vi "function2New.vi"   [LabVIEW 2016, in "Test.lvrbt"]
uses:
  Test.lvrbt
  <vilib>/NXT/Block Support/NXT_InputPort.ctl
  <vilib>/NXT/Hardware/Plugins/Tetrix DC Motor/TetrixDCMotorAddress.ctl
  <vilib>/NXT/NXTIO Xnodes/NXTIONodeSubVIs/TETRIX IO Move DC Motors.vi
  <vilib>/NXT/Dual Mode Library/Waits/Wait_EV3_Ultrasonic_Centimeter_Closer.vi
  <vilib>/NXT/NXTIO Xnodes/NXTIONodeSubVIs/TETRIX IO Stop DC Motors.vi
  <vilib>/NXT/Dual Mode Library/Waits/Wait_Num.vi
  <vilib>/NXT/Dual Mode Library/Waits/Wait_EV3_Ultrasonic_Centimeters_Further.vi
  <vilib>/NXT/Subs/LVHSConnector.ctl
  <vilib>/NXT/NXTIO Xnodes/AddressXNode/NXTIOAddress.xnode
  <vilib>/NXT/NXTIO Xnodes/NXTIOXNode/NXTIO.xnode
  <vilib>/NXT/LegoClasses/BrickReference/BrickReference.lvclass
types:
  T1 = typedef "NXT_InputPort.ctl" = u32
  T2 = typedef "TetrixDCMotorAddress.ctl" = i32
  T3 = typedef "LVHSConnector.ctl" = refnum<class "BrickReference.lvclass">
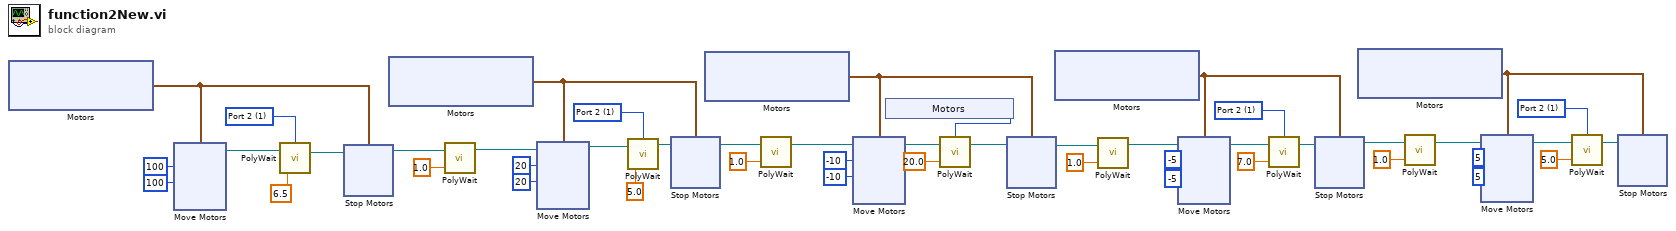
[diagram p0: block diagram]
diagram:
  w6 = T1 1 items=["Port 1", "Port 2", "Port 3", "Port 4"] ("Port (Port 1)")
  w13 = T1 1 items=["Port 1", "Port 2", "Port 3", "Port 4"] ("Port (Port 1)")
  w23 = T1 1 items=["Port 1", "Port 2", "Port 3", "Port 4"] ("Port (Port 1)")
  w24 = T1 1 items=["Port 1", "Port 2", "Port 3", "Port 4"] ("Port (Port 1)")
  n1 = xnode "Motors"() -> ("Motor"=w42:cluster{"TetrixDCMotor":T2, "TetrixDCMotor":T2})
  n2 = xnode "Move Motors"("Power/Speed 2"=i8 100, "Power/Speed 1"=i8 100, "Motors"=w42) -> ("NXT/EV3"=w45:T3)  [unwired: 1 in]
  n3 = call-poly <vilib>:"PolyWait.vi"("Centimeters (40)"=sgl 6.5, "NXT/EV3"=w45, "Port (Port 1)"=w24) -> ("NXT/EV3"=w43:T3)  [unwired: 1 in]
  n4 = xnode "Stop Motors"("Motors"=w42, "NXT/EV3"=w43) -> ("NXT/EV3"=w41:T3)
  n5 = xnode "Motors"() -> ("Motor"=w33:cluster{"TetrixDCMotor":T2, "TetrixDCMotor":T2})
  n6 = call-poly <vilib>:"PolyWait.vi"("Time (1 sec)"=sgl 1.0, "NXT/EV3"=w41) -> ("NXT/EV3"=w39:T3)  [unwired: 2 in]
  n7 = xnode "Move Motors"("Power/Speed 2"=i8 20, "Power/Speed 1"=i8 20, "Motors"=w33, "NXT/EV3"=w39) -> ("NXT/EV3"=w36:T3)
  n8 = call-poly <vilib>:"PolyWait.vi"("Centimeters (50)"=sgl 5.0, "NXT/EV3"=w36, "Port (Port 1)"=w23) -> ("NXT/EV3"=w34:T3)  [unwired: 1 in]
  n9 = xnode "Stop Motors"("Motors"=w33, "NXT/EV3"=w34) -> ("NXT/EV3"=w30:T3)
  n10 = xnode "Motors"() -> ("Motor"=w25:cluster{"TetrixDCMotor":T2, "TetrixDCMotor":T2})
  n11 = call-poly <vilib>:"PolyWait.vi"("Time (1 sec)"=sgl 1.0, "NXT/EV3"=w30) -> ("NXT/EV3"=w29:T3)  [unwired: 2 in]
  n12 = xnode "Move Motors"("Power/Speed 2"=i8 -10, "Power/Speed 1"=i8 -10, "Motors"=w25, "NXT/EV3"=w29) -> ("NXT/EV3"=w28:T3)
  n13 = xnode "Motors"() -> ("Sensor"=w21:T1)
  n14 = call-poly <vilib>:"PolyWait.vi"("Centimeters (40)"=sgl 20.0 ("Time (1 sec)"), "NXT/EV3"=w28, "Port (Port 1)"=w21) -> ("NXT/EV3"=w26:T3)  [unwired: 1 in]
  n15 = xnode "Stop Motors"("Motors"=w25, "NXT/EV3"=w26) -> ("NXT/EV3"=w19:T3)
  n16 = xnode "Motors"() -> ("Motor"=w11:cluster{"TetrixDCMotor":T2, "TetrixDCMotor":T2})
  n17 = call-poly <vilib>:"PolyWait.vi"("Time (1 sec)"=sgl 1.0, "NXT/EV3"=w19) -> ("NXT/EV3"=w18:T3)  [unwired: 2 in]
  n18 = xnode "Move Motors"("Power/Speed 2"=i8 -5, "Power/Speed 1"=i8 -5, "Motors"=w11, "NXT/EV3"=w18) -> ("NXT/EV3"=w14:T3)
  n19 = call-poly <vilib>:"PolyWait.vi"("Centimeters (40)"=sgl 7.0 ("Time (1 sec)"), "NXT/EV3"=w14, "Port (Port 1)"=w13) -> ("NXT/EV3"=w12:T3)  [unwired: 1 in]
  n20 = xnode "Stop Motors"("Motors"=w11, "NXT/EV3"=w12) -> ("NXT/EV3"=w2:T3)
  n21 = xnode "Motors"() -> ("Motor"=w4:cluster{"TetrixDCMotor":T2, "TetrixDCMotor":T2})
  n22 = call-poly <vilib>:"PolyWait.vi"("Time (1 sec)"=sgl 1.0, "NXT/EV3"=w2) -> ("NXT/EV3"=w1:T3)  [unwired: 2 in]
  n23 = xnode "Move Motors"("Power/Speed 2"=i8 5, "Power/Speed 1"=i8 5, "Motors"=w4, "NXT/EV3"=w1) -> ("NXT/EV3"=w7:T3)
  n24 = call-poly <vilib>:"PolyWait.vi"("Centimeters (50)"=sgl 5.0 ("Time (1 sec)"), "NXT/EV3"=w7, "Port (Port 1)"=w6) -> ("NXT/EV3"=w5:T3)  [unwired: 1 in]
  n25 = xnode "Stop Motors"("Motors"=w4, "NXT/EV3"=w5) -> ()  [unwired: 1 out]
